vi "TreeNode Put Segment.vi"(8 "error in (no error)":errorcluster, 9 "Offset (-1)":i32=-1, 10 "Data":refnum<data-value>, 11 "TreeNode DVR in":refnum<data-value>) -> (0 "error out":errorcluster, 3 "TreeNode DVR out":refnum<data-value>)   [LabVIEW 2012, in "MDSplus.lvlib"]
doc: "Write (part of) data segment."
uses:
  <vilib>/MDSplus/Library/MDSplus.lvlib
  <vilib>/MDSplus/Classes/Data_Class/TreeNode_Class/TreeNode.lvclass
  <vilib>/MDSplus/Classes/Data_Class/Array_Class/Array.lvclass
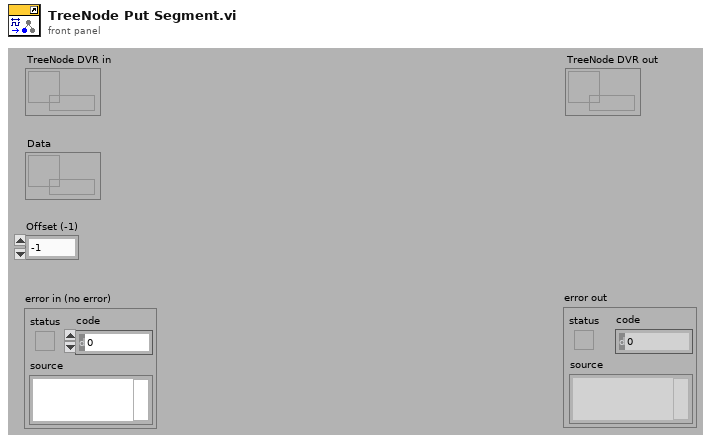
[diagram p1: front panel]
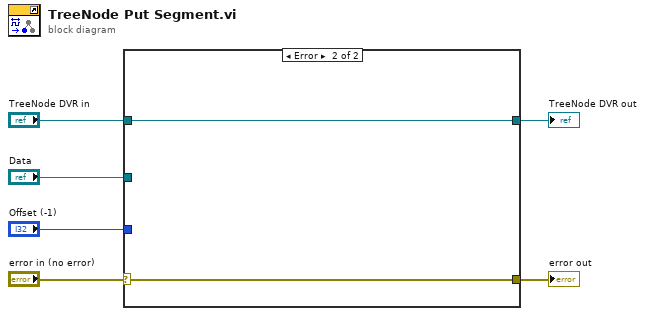
[diagram p0: block diagram]
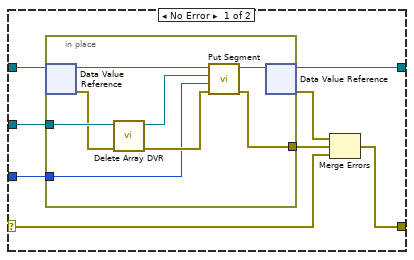
[diagram p2: hidden frame]
diagram:
  n1 = case shown="Error" "error in (no error)" {
    selector: "error in (no error)" -> [w13 w23]
    tunnel: "TreeNode DVR in" -> [w14 w24]
    tunnel: [w10 w23] -> w6
    tunnel: [w11 w24] -> w3
    tunnel: "Data" -> [w8 _]
    tunnel: "Offset (-1)" -> [w7 _]
    frame No Error {
      n2 = in-place {
        in-place-border: [w16] -> w9
        in-place-border: w8 -> [w20]
        in-place-border: w7 -> [w15]
        n3 = in-place-dvr #1(w14) -> (w22:refnum<class "TreeNode.lvclass">, w19:errorcluster)
        n4 = call <vilib>:"Delete Array DVR.vi"("error in (no error)"=w19, "Array DVR in"=w20) -> ("error out"=w18:errorcluster, "Array out"=w17:refnum<class "Array.lvclass">)  [unwired: 8 in]
        n5 = call-dynamic "Put Segment.vi"("error in (no error)"=w18, "Offset (-1)"=w15, "Data"=w17, "TreeNode in"=w22) -> ("error out"=w16:errorcluster, "TreeNode out"=w21:refnum<class "TreeNode.lvclass">)  [unwired: 6 in]
        n6 = in-place-dvr #1(w21) -> (w11:refnum<data-value>, w12:errorcluster)
      }
      n7 = Merge Errors(w12, w9, w13) -> (w10:errorcluster)
    }
    frame Error {
    }
  }
  "error out" <- w6
  "TreeNode DVR out" <- w3
